vi "Instantiate.vi"(8 "error in (no error)":errorcluster, 10 "gRPCid":T1, 11 "iService":refnum<class "iService.lvclass">) -> (0 "error out":errorcluster, 3 "iService":refnum<class "iService.lvclass">)   [LabVIEW 2019, in "gRPC-servicer.lvlib" / "iService.lvclass"]
uses:
  iService.lvclass
  <vilib>/gRPC/LabVIEW gRPC Library/Server API/typeDefs/grpcId.ctl
  iService.lvclass/iService.ctl
  <vilib>/gRPC/LabVIEW gRPC Library/gprc-lvsupport-release.lvlib
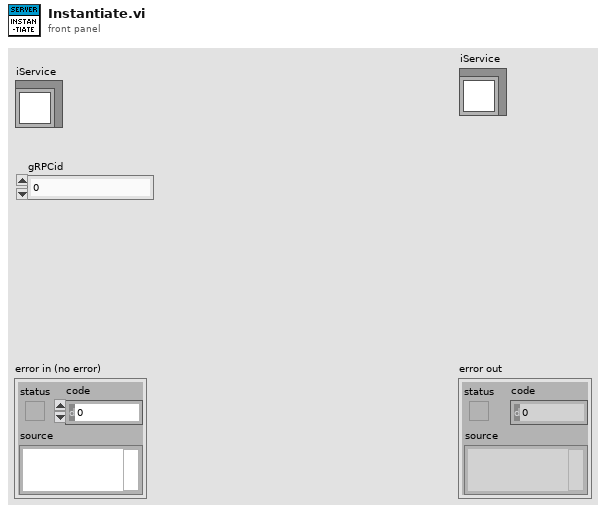
[diagram p1: front panel]
types:
  T1 = typedef "gprc-lvsupport-release.lvlib/grpcId.ctl" = u64
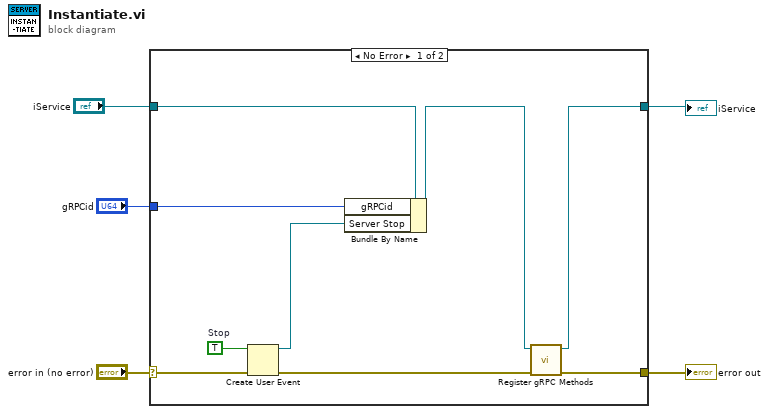
[diagram p0: block diagram]
diagram:
  n1 = case shown="No Error" "error in (no error)" {
    selector: "error in (no error)" -> [w14 w16]
    tunnel: [w9 w16] -> w4
    tunnel: [w7 w15] -> w3
    tunnel: "gRPCid" -> [w6 _]
    tunnel: "iService" -> [w11 w15]
    frame No Error {
      w13 = TRUE  # Stop
      n2 = Create User Event(user event datatype=w13, error in=w14) -> (user event=w12:refnum<user-event>, error out=w10:errorcluster)
      n3 = Bundle By Name(cluster=w11, "gRPCid"=w6, "Server Stop"=w12) -> (w8:refnum<class "iService.lvclass">)
      n4 = call-dynamic "Register gRPC Methods.vi"("error in (no error)"=w10, "Template Server in"=w8) -> ("error out"=w9:errorcluster, "Template Server out"=w7:refnum<class "iService.lvclass">)  [unwired: 8 in]
    }
    frame Error {
    }
  }
  "error out" <- w4
  "iService" <- w3
